vi "Main.vi"(8 "error in (no error)":errorcluster, 11 "ModuleAdmin":refnum<class "ModuleAdmin.lvclass">) -> ()   [LabVIEW 2018, in "ScopePlugins.lvlib"]
uses:
  ScopePlugins.lvlib
  <userlib>/NIST/ModuleAdminLib/ModuleAdmin/ModuleAdmin.lvclass
  C:/Program Files (x86)/National Instruments/LabVIEW 2018/user.lib/NIST/ModuleAdminLib/ModuleAdminBase/ModuleAdminBase.lvclass
  Shared/TypeDefs/QueueNames.ctl
  ScopePluginBaseClass/ScopePluginsBase.lvclass
  C:/Program Files (x86)/National Instruments/LabVIEW 2018/user.lib/NIST/BaseClasses/BasePlugin_class/BasePlugin.lvclass
  Shared/Queue&Messages/EnqueueTypes.ctl
  Shared/Queue&Messages/DequeueTypes.ctl
  ScopeShared/clStopArgument.ctl
  <userlib>/NIST/ModuleAdminLib/ModuleAdmin/ModuleAdmin.lvclass/ModuleAdmin.ctl
  ScopePluginBaseClass/ScopePluginsBase.lvclass/ScopePluginsBase.ctl
  <userlib>/NIST/BaseClasses/BasePlugin_class/BasePlugin.lvclass/BasePlugin.ctl
  InfiniiumClass/Typedefs/ExtAcquisition.ctl
  ScopeShared/Sync.ctl
  <vilib>/Utility/error.llb/DialogType.ctl
  <userlib>/NIST/ModuleAdminLib/ModuleAdmin/Accessors/Read ShowPanel_.vi
  ScopePluginBaseClass/Accessors/Write ModuleID.vi
  ScopePluginBaseClass/Accessors/Read ModuleID.vi
  <userlib>/NIST/ModuleAdminLib/ModuleAdmin/Accessors/Write ShowPanel_.vi
  <userlib>/NIST/BaseClasses/BasePlugin_class/Accessors/Read PluginIniFilePath.vi
  ScopePluginBaseClass/Accessors/Write Sync.vi
  <userlib>/NIST/ModuleAdminLib/ModuleAdmin/Accessors/Read CloneRegRef.vi
  <extravilib>/ChannelInstances/Tag-bool/Read With Abort.vi
  <extravilib>/ChannelInstances/Tag-bool/Write With Abort.vi
  <extravilib>/ChannelInstances/Tag-bool/Instantiate.vi
  <extravilib>/ChannelInstances/Tag-bool/EndpointRead.vi
  <vilib>/Utility/error.llb/Error Cluster From Error Code.vi
  <extravilib>/ChannelInstances/Tag-bool/Endpoint.vi
  <vilib>/ErrorRing/Error Ring.xnode
  <userlib>/NIST/ModuleAdminLib/CloneRegistration/CloneRegistration.lvclass
  ScopeShared/ScopeShared.lvlib
  <userlib>/NIST/ModuleAdminLib/ModuleAdmin.lvlib
  <userlib>/NIST/BaseClasses/Object_class/BaseObject.lvclass
  InfiniiumClass/Infiniium.lvclass
  <extravilib>/ChannelInstances/Tag-bool.lvlib
panel:
  out "EH Loop":i32
  out "QMH Loop":i32
  out "WA Loop":i32
  out "error out":errorcluster
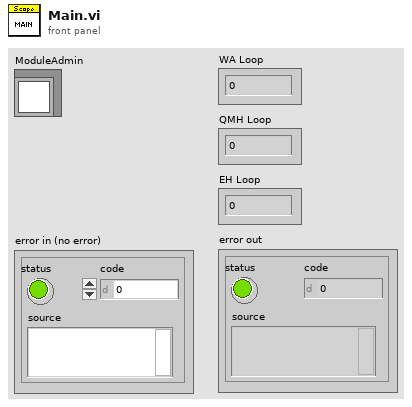
[diagram p1: front panel]
types:
  T1 = typedef "ScopePlugins.lvlib/EnqueueTypes.ctl" = enum16{"LossyEnqueue", "EnqueueAtFront", "Enqueue"}
  T2 = typedef "ScopePlugins.lvlib/QueueNames.ctl" = enum16{"QMH", "Class ", "MA"}
  T3 = typedef "ScopeShared.lvlib/clRequestEvents.ctl" = cluster{"StopRequest":refnum<user-event>, "PathToINI":refnum<user-event>, " LoadPlugin":refnum<user-event>, "ShowPanel":refnum<user-event>, "Abort":refnum<user-event>, "SetAcquisition":refnum<user-event>, "SetChannel":refnum<user-event>, "SetTrigger":refnum<user-event>, "GetAcquisition":refnum<user-event>, "GetChannel":refnum<user-event>, "GetTrigger":refnum<user-event>, "FetchWaveform":refnum<user-event>, "InitAcquisition":refnum<user-event>, "ReadWaveform":refnum<user-event>, "GetHandle":refnum<user-event>, "SetHandle":refnum<user-event>, "GetModel":refnum<user-event>, "SetModel":refnum<user-event>, "ConfigAquisition":refnum<user-event>, "ConfigChannels":refnum<user-event>, "ConfigTrigger":refnum<user-event>, "Initialize":refnum<user-event>, "SetExtAcquisition":refnum<user-event>, "StopAcquisition":refnum<user-event>, "PrefDlg":refnum<user-event>, "Close":refnum<user-event>, "SetSync":refnum<user-event>}
  T4 = typedef "ScopeShared.lvlib/clBroadcastEvents.ctl" = cluster{"DidInit":refnum<user-event>, "StatusUpdate":refnum<user-event>, "ErrorReport":refnum<user-event>, "DidStop":refnum<user-event>, "PathToINI":refnum<user-event>, "Handle":refnum<user-event>, "Model":refnum<user-event>, "Channels":refnum<user-event>, "Acquisition":refnum<user-event>, "Trigger":refnum<user-event>, "ExtAcquisition":refnum<user-event>, "Waveform":refnum<user-event>}
  T5 = typedef "ScopePlugins.lvlib/DequeueTypes.ctl" = enum16{"PreviewQueue", "Dequeue"}
  T6 = typedef "ScopeShared.lvlib/clStopArgument.ctl" = cluster{"Exit via Stop Module Req?":bool, "Wait for Module to stop?":bool, "ModuleAdmin":refnum<class "ModuleAdmin.lvclass">}
  T7 = enum32{"Invalid", "Standard", "Closed", "Hidden", "Minimized", "Maximized"}
  T8 = typedef "ScopePlugins.lvlib/Infiniium.lvclass/ExtAcquisition.ctl" = cluster{"SamplingMode ":enum16{"Real Time", "Equivalent Time", "Segment", "Real Time Peak Detect", "Real Time High Resolution", "Peak Detect Segment", "High Resolution Segment"}, "Interpolation":enum16{"No Interpolation", "sin(x)/x", "linear", "1 Point sin(x)/x", "2 Point sin(x)/x", "4 Point sin(x)/x", "8 Point sin(x)/x", "16 Point sin(x)/x"}, "NumAverages":i32, "EnableAveraging":bool, "Resolution":enum16{"Auto", "Bits 9", "Bits 10", "Bits 11", "Bits 12"}}
  T9 = typedef "ScopeShared.lvlib/Sync.ctl" = cluster{"Handle":string, "SrcTerm":string, "DestTerm":string}
  T10 = typedef "ScopeShared.lvlib/Waveform.ctl" = cluster{"initial x":dbl, "x increment":dbl, "waveform array":dbl[]}
  T11 = typedef "Tag-bool.lvlib/))Channel.ctl" = refnum<queue>
  T12 = typedef "DialogType.ctl" = u16
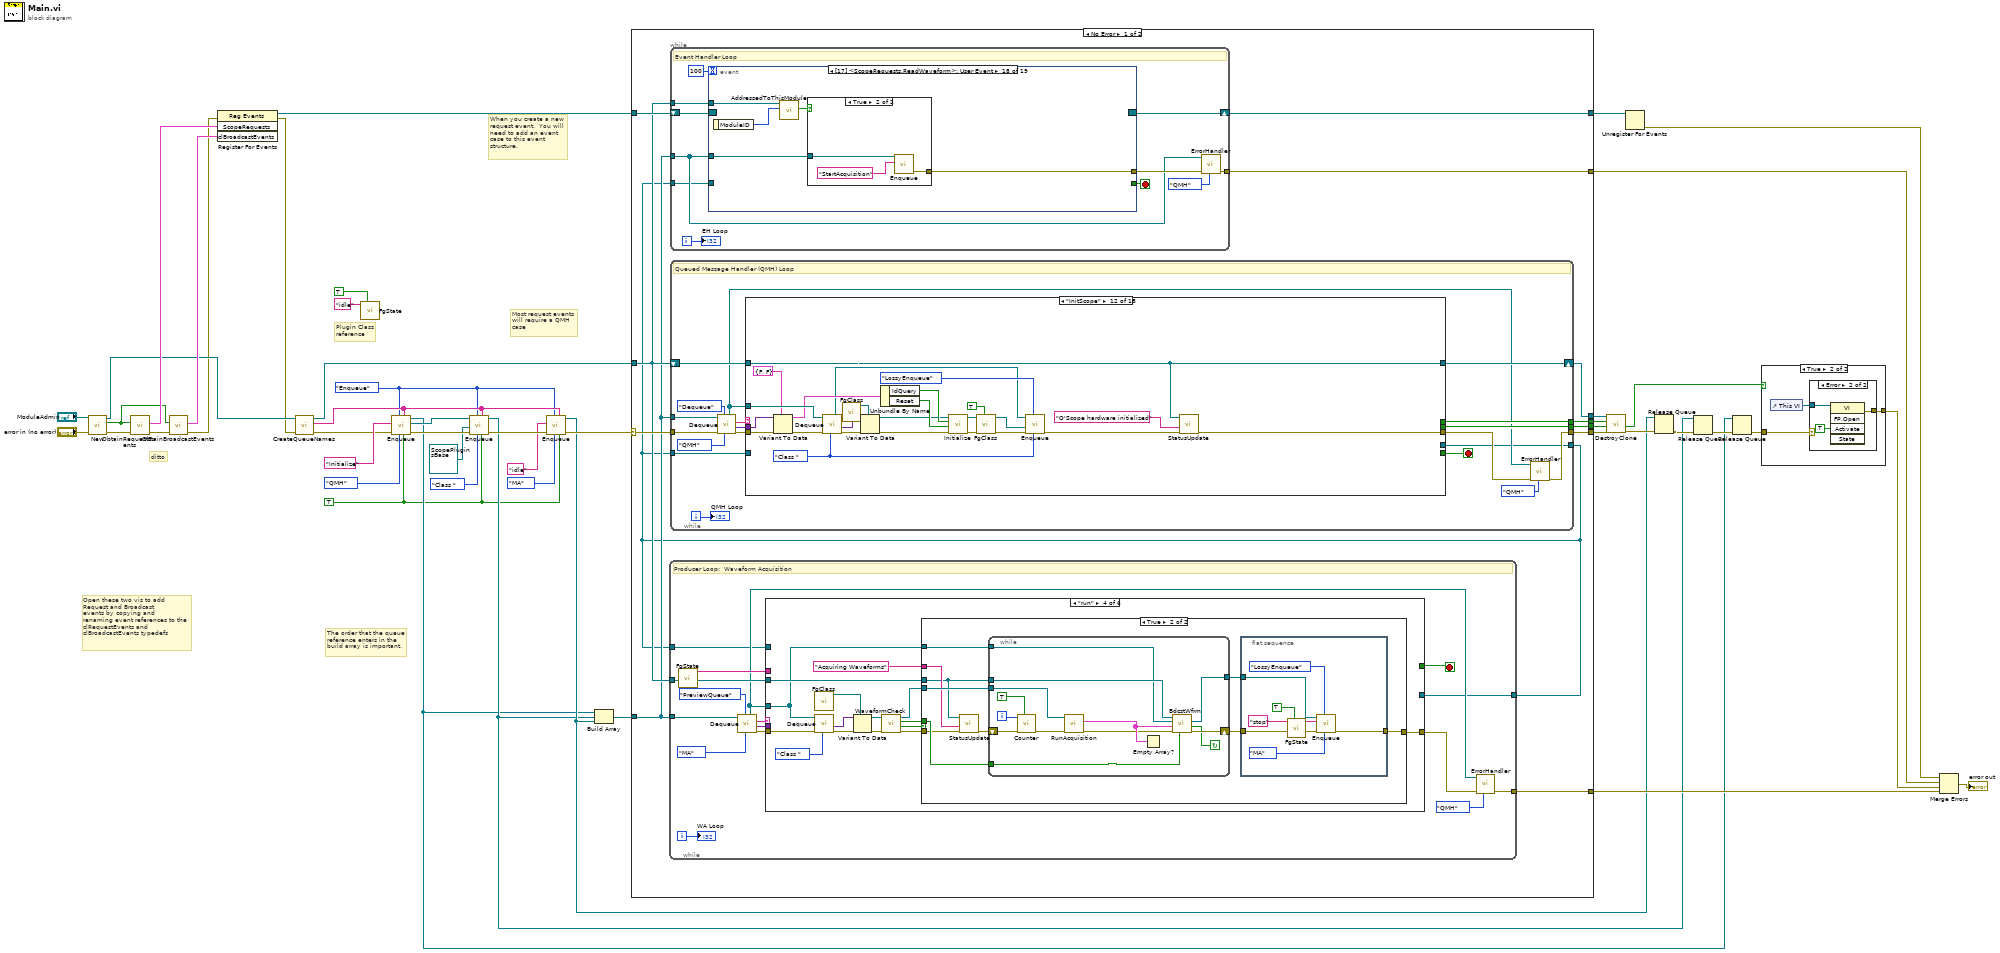
[diagram p0: block diagram]
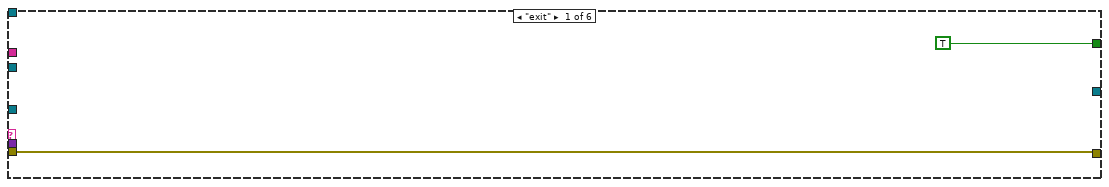
[diagram p2: hidden frame]
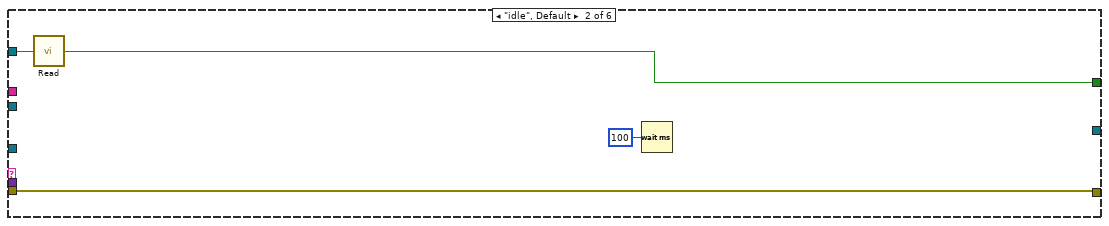
[diagram p3: hidden frame]
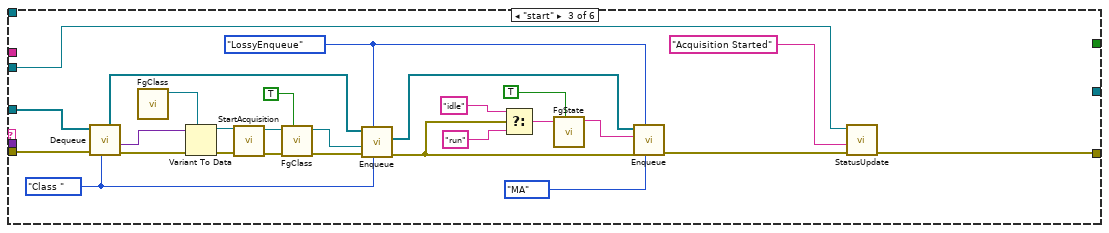
[diagram p4: hidden frame]
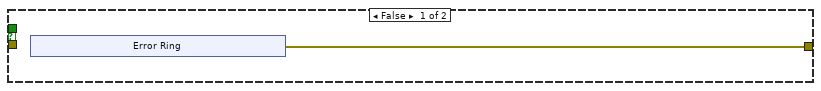
[diagram p5: hidden frame]
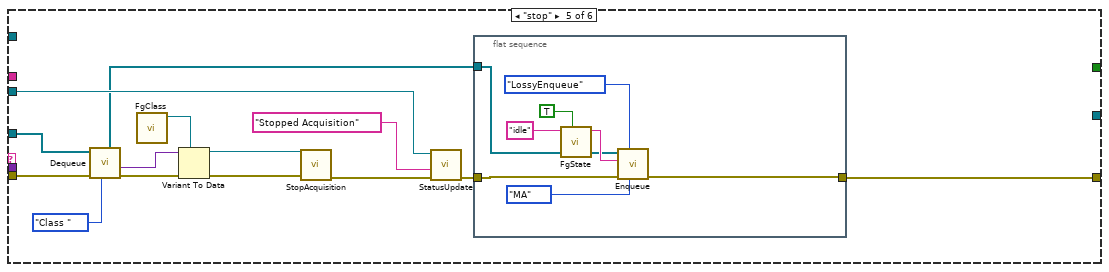
[diagram p6: hidden frame]
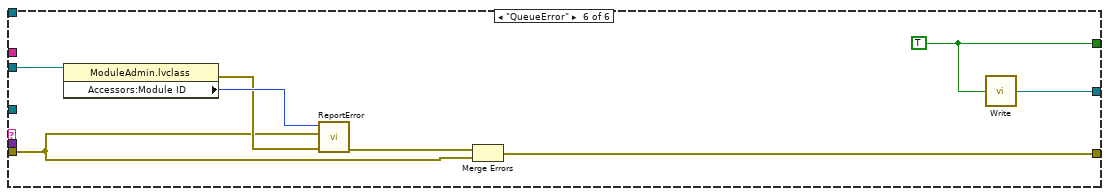
[diagram p7: hidden frame]
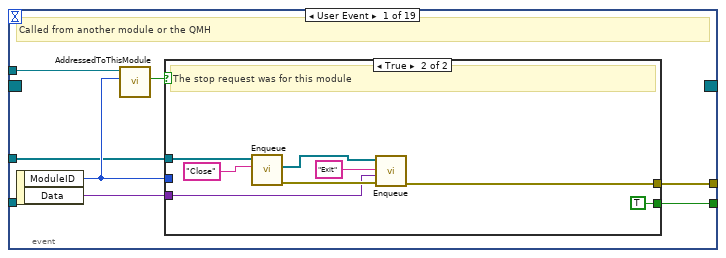
[diagram p8: hidden frame]
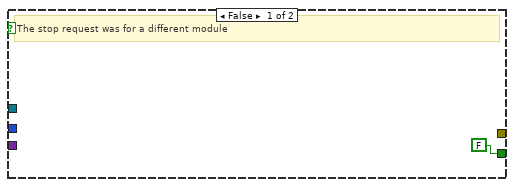
[diagram p9: hidden frame]
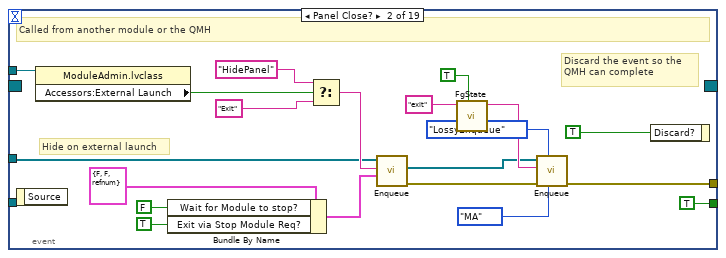
[diagram p10: hidden frame]
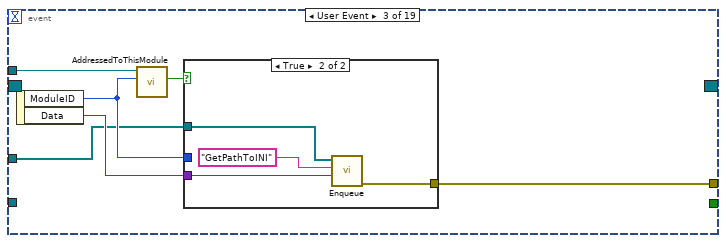
[diagram p11: hidden frame]
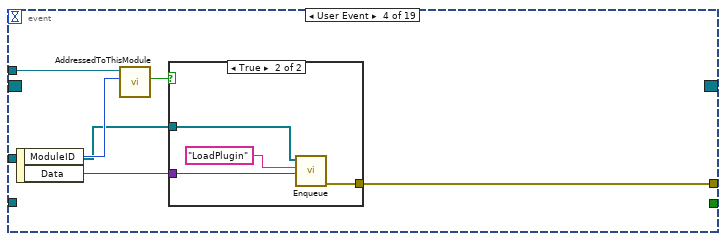
[diagram p13: hidden frame]
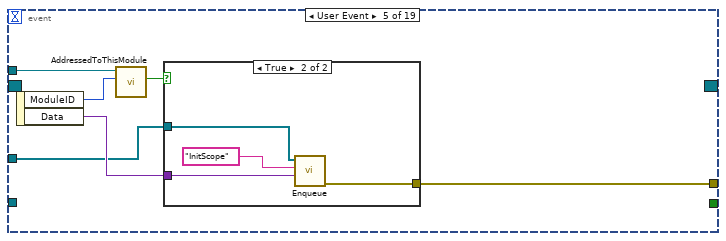
[diagram p15: hidden frame]
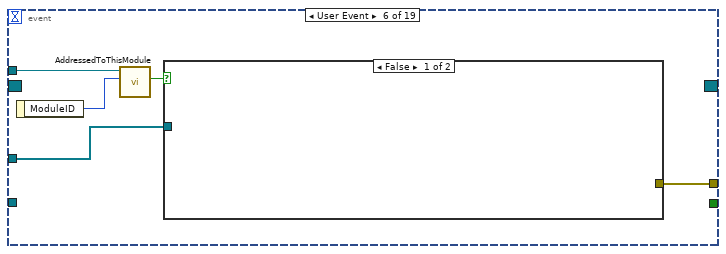
[diagram p17: hidden frame]
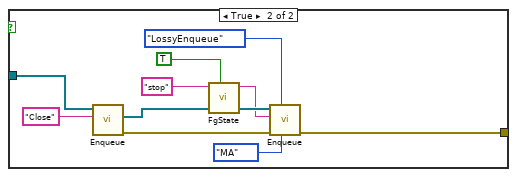
[diagram p18: hidden frame]
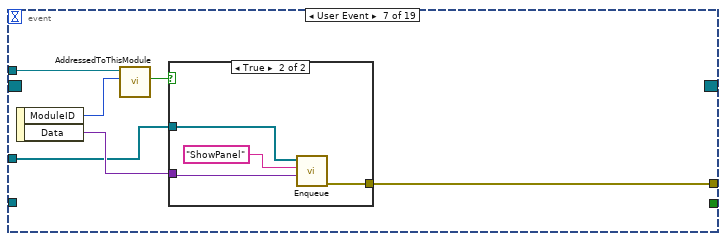
[diagram p19: hidden frame]
diagram:
  w3 = EnqueueTypes."Enqueue" ("EnqueueType (Enqueue)")
  w4 = TRUE ("Frist Call (F)")
  # "The order that the queue\nreference enters in the \nbuild array is important."
  # "Plugin Class\nreference"
  # "Open these two vis to add\nRequest and Broadcast \nevents by copying and \nrenaming event references to the \nclRequestEvents and \nclBroadcastEvents typedefs"
  # "ditto"
  # "Most request events\nwill require a QMH\ncase"
  # "When you create a new request event.  You will need to add an event case to this event structure."
  n1 = call <userlib>:"New.vi"("error in (no error)"="error in (no error)", "ModuleAdmin"="ModuleAdmin") -> ("error out"=w45:errorcluster, "First?"=w43:bool, "ModuleAdmin"=w28:refnum<class "ModuleAdmin.lvclass">)  [unwired: 6 in, 1 out]
  n2 = call "ObtainRequestEvents.vi"("error in (no error)"=w45, "CreateNew (F)"=w43) -> ("error out"=w42:errorcluster, "ScopeRequests"=w44:T3)  [unwired: 8 in]
  n3 = call "ObtainBroadcastEvents.vi"("error in (no error)"=w42, "CreateNew? (F)"=w43) -> ("error out"=w25:errorcluster, "clBroadcastEvents"=w41:T4)  [unwired: 8 in]
  n4 = register-events(error in=w25, w44, w41) -> (reference out=w40:refnum<event-registration>, error out=w26:errorcluster)  [unwired: 1 in]
  n5 = call "CreateQueueNames.vi"("error in (no error)"=w26, "ModuleAdmin In"=w28) -> ("error out"=w19:errorcluster, "QueueNames Out"=w9:string[], "ModuleAdmin Out"=w27:refnum<class "ModuleAdmin.lvclass">)  [unwired: 7 in]
  n6 = call "FgState.vi"("Set (F)"=TRUE, "State In"="idle") -> ()  [unwired: 9 in, 1 out]
  n7 = call "Enqueue.vi"("Frist Call (F)"=w4, "QueueNames In"=w9, "EnqueueType (QMH)"=QueueNames."QMH", "EnqueueType (Enqueue)"=w3, "error in (no error)"=w19, "Message"="Initialize") -> ("error out"=w18:errorcluster, "Queue Array Reference Out"=w16:refnum<queue>[], "MessageQueue"=w6:refnum<queue>)  [unwired: 3 in]
  n8 = call "Enqueue.vi"("Frist Call (F)"=w4, "QueueNames In"=w9, "EnqueueType (QMH)"=QueueNames."Class ", "EnqueueType (Enqueue)"=w3, "error in (no error)"=w18, "Message Data"=refnum<class "ScopePluginsBase.lvclass"> refnum ("MyPlugins.lvlib:MyPluginsBase.lvclass"), "Queue Array Reference In"=w16) -> ("error out"=w15:errorcluster, "MessageQueue"=w7:refnum<queue>)  [unwired: 2 in, 1 out]
  n9 = call "Enqueue.vi"("Frist Call (F)"=w4, "QueueNames In"=w9, "EnqueueType (QMH)"=QueueNames."MA", "EnqueueType (Enqueue)"=w3, "error in (no error)"=w15, "Message"="idle") -> ("error out"=w14:errorcluster, "MessageQueue"=w8:refnum<queue>)  [unwired: 3 in, 1 out]
  n10 = Build Array(w6, w7, w8) -> (w5:refnum<queue>[])
  n11 = case shown="No Error" w14 {
    selector: w14 -> [w52 w773]
    tunnel: w27 -> [w51 w771]
    tunnel: [w59 w767] -> w39
    tunnel: w40 -> [w58 w766]
    tunnel: [w57 w770] -> w37
    tunnel: [w56 _] -> w36
    tunnel: [w55 _] -> w35
    tunnel: [w54 w767] -> w11
    tunnel: [w53 w767] -> w30
    tunnel: w5 -> [w50 _]
    tunnel: [w48 w766] -> w2
    frame No Error {
      n12 = while {
        tunnel: [w72] -> w53
        tunnel: w50 -> [w67]
        tunnel: w51 -> [w64]
        tunnel: [w61] -> w49
        tunnel: w49 -> [w60]
        i -> [w63]
        stop <- w74 stop-if-true
        # "Producer Loop:  Waveform Acquisition"
        n13 = call "FgState.vi"() -> ("State Out"=w75:string)  [unwired: 11 in]
        n14 = call "Dequeue.vi"("EnqueueType (QMH)"=QueueNames."MA", "DequeueType (PreviewQueue)"=DequeueTypes."PreviewQueue", "Queue Array Reference In"=w67) -> ("error out"=w71:errorcluster, "Message Data"=w69:variant, "Message"=w70:string, "Queue Array Reference Out"=w62:refnum<queue>[])  [unwired: 4 in, 1 out]
        n15 = case shown="\"run\"" w70 {
          tunnel: [TRUE w78 _ _ _ w183] -> w74
          tunnel: [w76 w80 w82 w122 w170 w184] -> w73
          tunnel: w71 -> [w76 w80 w100 w112 w168 w186]
          tunnel: w69 -> [_ _ _ _ _ _]
          tunnel: w64 -> [_ _ w83 w121 w169 w185]
          tunnel: w75 -> [_ _ _ _ _ _]
          tunnel: w62 -> [_ _ w87 w108 w161 _]
          tunnel: [_ _ _ _ _ w182] -> w61
          tunnel: w60 -> [_ w79 _ _ _ _]
          frame "exit" {
          }
          frame "idle", Default {
            n16 = call <extravilib>:"Read.vi"("channel"=w79) -> ("element"=w78:bool)  [unwired: 1 in, 1 out]
            n17 = Wait (ms)(milliseconds to wait=u32 100) -> ()  [unwired: 1 out]
          }
          frame "start" {
            w98 = QueueNames."Class " ("EnqueueType (QMH)")
            w86 = EnqueueTypes."LossyEnqueue" ("EnqueueType (Enqueue)")
            n18 = call "Dequeue.vi"("EnqueueType (QMH)"=w98, "error in (no error)"=w100, "Queue Array Reference In"=w87) -> ("error out"=w103:errorcluster, "Message Data"=w102:variant, "Queue Array Reference Out"=w88:refnum<queue>[])  [unwired: 4 in, 2 out]
            n19 = call "FgClass.vi"() -> ("Class Out"=w101:refnum<class "ScopePluginsBase.lvclass">)  [unwired: 11 in]
            n20 = Variant To Data(error in=w103, type=w101, Variant=w102) -> (data=w97:refnum<class "ScopePluginsBase.lvclass">, error out=w99:errorcluster)
            n21 = call-dynamic "StartAcquisition.vi"("error in (no error)"=w99, "ScopePluginsBase in"=w97) -> ("error out"=w104:errorcluster, "ScopePluginsBase out"=w90:refnum<class "ScopePluginsBase.lvclass">)  [unwired: 8 in]
            n22 = call "FgClass.vi"("Set (F)"=TRUE, "Class In"=w90) -> ("Class Out"=w89:refnum<class "ScopePluginsBase.lvclass">)  [unwired: 9 in]
            n23 = call "Enqueue.vi"("EnqueueType (QMH)"=w98, "EnqueueType (Enqueue)"=w86, "error in (no error)"=w104, "Message Data"=w89, "Queue Array Reference In"=w88) -> ("error out"=w96:errorcluster, "Queue Array Reference Out"=w95:refnum<queue>[])  [unwired: 4 in, 1 out]
            n24 = Select(t="idle" ("State In"), s=w96, f="run") -> (s? t:f=w94:string)
            n25 = call "FgState.vi"("Set (F)"=TRUE, "State In"=w94) -> ("State Out"=w92:string)  [unwired: 9 in]
            n26 = call "Enqueue.vi"("EnqueueType (QMH)"=QueueNames."MA", "EnqueueType (Enqueue)"=w86, "error in (no error)"=w96, "Message"=w92, "Queue Array Reference In"=w95) -> ("error out"=w84:errorcluster)  [unwired: 4 in, 2 out]
            n27 = call "StatusUpdate.vi"("error in (no error)"=w84, "Status"="Acquisition Started", "ModuleAdmin"=w83) -> ("error out"=w82:errorcluster)  [unwired: 8 in]
          }
          frame "run" {
            n28 = call "FgClass.vi"() -> ("Class Out"=w110:refnum<class "ScopePluginsBase.lvclass">)  [unwired: 11 in]
            n29 = call "Dequeue.vi"("EnqueueType (QMH)"=QueueNames."Class ", "error in (no error)"=w112, "Queue Array Reference In"=w108) -> ("error out"=w115:errorcluster, "Message Data"=w114:variant)  [unwired: 4 in, 3 out]
            n30 = Variant To Data(error in=w115, type=w110, Variant=w114) -> (data=w109:refnum<class "ScopePluginsBase.lvclass">, error out=w111:errorcluster)
            n31 = call "WaveformCheck.vi"("error in (no error)"=w111, "Class In"=w109) -> ("error out"=w116:errorcluster, "Run?"=w118:bool, "Continuous"=w119:bool, "Class Out"=w117:refnum<class "ScopePluginsBase.lvclass">)  [unwired: 6 in]
            n32 = case shown="True" w118 {
              tunnel: [w123 w136] -> w122
              tunnel: w117 -> [_ w138]
              tunnel: w119 -> [_ w137]
              tunnel: w116 -> [_ w135]
              tunnel: w121 -> [_ w131]
              tunnel: "Acquiring Waveforms" ("Status") -> [_ w132]
              tunnel: w108 -> [_ w130]
              frame False {
                n33 = xnode "Error Ring"() -> ("error out"=w123:errorcluster)
              }
              frame True {
                n34 = call "StatusUpdate.vi"("error in (no error)"=w135, "Status"=w132, "ModuleAdmin"=w131) -> ("error out"=w134:errorcluster)  [unwired: 8 in]
                n35 = while {
                  tunnel: w138 -> [w151]
                  tunnel: w137 -> [w139]
                  shift-right: [w150] -> w133
                  shift-left: w134 -> [w148]
                  tunnel: w131 -> [w144]
                  tunnel: w130 -> [w141]
                  tunnel: [w143] -> w129
                  i -> [w146]
                  stop <- w140 continue-if-true
                  n36 = call "Counter.vi"("Set (f)"=TRUE, "error in (no error)"=w148, "Counter In"=w146) -> ("error out"=w147:errorcluster)  [unwired: 7 in, 1 out]
                  n37 = call-dynamic "RunAcquisition.vi"("error in (no error)"=w147, "ScopePluginsBase in"=w151) -> ("error out"=w142:errorcluster, "Waveforms"=w149:T10[])  [unwired: 7 in, 1 out]
                  n38 = Empty Array?(array=w149) -> ()  [unwired: 1 out]
                  n39 = call "BdcstWfrm.vi"("Continuous"=w139, "error in (no error)"=w142, "Waveforms"=w149, "Queue Array Reference In"=w141, "ModuleAdmin"=w144) -> ("error out"=w150:errorcluster, "Continue"=w140:bool, "Queue Array Reference Out"=w143:refnum<queue>[])  [unwired: 4 in]
                }
                n40 = flat-sequence {
                  tunnel: w133 -> [w156]
                  tunnel: [w155] -> w136
                  tunnel: w129 -> [w152]
                  frame #0 {
                    n41 = call "FgState.vi"("Set (F)"=TRUE, "State In"="stop") -> ("State Out"=w153:string)  [unwired: 9 in]
                    n42 = call "Enqueue.vi"("EnqueueType (QMH)"=QueueNames."MA", "EnqueueType (Enqueue)"=EnqueueTypes."LossyEnqueue", "error in (no error)"=w156, "Message"=w153, "Queue Array Reference In"=w152) -> ("error out"=w155:errorcluster)  [unwired: 4 in, 2 out]
                  }
                }
              }
            }
          }
          frame "stop" {
            n43 = call "Dequeue.vi"("EnqueueType (QMH)"=QueueNames."Class ", "error in (no error)"=w168, "Queue Array Reference In"=w161) -> ("error out"=w167:errorcluster, "Message Data"=w166:variant, "Queue Array Reference Out"=w160:refnum<queue>[])  [unwired: 4 in, 2 out]
            n44 = call "FgClass.vi"() -> ("Class Out"=w163:refnum<class "ScopePluginsBase.lvclass">)  [unwired: 11 in]
            n45 = Variant To Data(error in=w167, type=w163, Variant=w166) -> (data=w162:refnum<class "ScopePluginsBase.lvclass">, error out=w165:errorcluster)
            n46 = call-dynamic "StopAcquisition.vi"("error in (no error)"=w165, "ScopePluginsBase in"=w162) -> ("error out"=w172:errorcluster)  [unwired: 8 in, 1 out]
            n47 = call "StatusUpdate.vi"("error in (no error)"=w172, "Status"="Stopped Acquisition", "ModuleAdmin"=w169) -> ("error out"=w171:errorcluster)  [unwired: 8 in]
            n48 = flat-sequence {
              tunnel: w171 -> [w179]
              tunnel: [w178] -> w170
              tunnel: w160 -> [w174]
              frame #0 {
                n49 = call "FgState.vi"("Set (F)"=TRUE, "State In"="idle") -> ("State Out"=w175:string)  [unwired: 9 in]
                n50 = call "Enqueue.vi"("EnqueueType (QMH)"=QueueNames."MA", "EnqueueType (Enqueue)"=EnqueueTypes."LossyEnqueue", "error in (no error)"=w179, "Message"=w175, "Queue Array Reference In"=w174) -> ("error out"=w178:errorcluster)  [unwired: 4 in, 2 out]
              }
            }
          }
          frame "QueueError" {
            w183 = TRUE ("Boolean")
            n51 = property class="ModuleAdmin.lvclass"(reference=w185) -> (error out=w188:errorcluster, "Accessors:Module ID"=w189:i32)  [unwired: 1 in, 1 out]
            n52 = call "ReportError.vi"("error in (no error)"=w188, "ErrorReported"=w186, "ModuleID"=w189) -> ("error out"=w187:errorcluster)  [unwired: 8 in]
            n53 = Merge Errors(w187, w186) -> (w184:errorcluster)
            n54 = call <extravilib>:"Write.vi"("element"=w183) -> ("channel"=w182:T11)  [unwired: 1 out]
          }
        }
        n55 = call "ErrorHandler.vi"("EnqueueType (QMH)"=QueueNames."QMH", "error in (no error)"=w73, "Queue Array Reference In"=w62) -> ("error out"=w72:errorcluster)  [unwired: 8 in]
        "WA Loop" <- w63
      }
      n56 = while {
        shift-right: [w198] -> w48
        shift-left: w58 -> [w199]
        tunnel: w51 -> [w197]
        tunnel: [w195] -> w54
        tunnel: w50 -> [w194]
        tunnel: w49 -> [w190]
        i -> [w192]
        stop <- w200 stop-if-true
        # "Event Handler Loop"
        n57 = event shown="[17] <ScopeRequests.ReadWaveform>: User Event" {
          selector: w199 -> [_ _ _ _ _ _ _ _ _ _ _ _ _ _ _ _ _ _ _]
          dyn-events: [_ _ _ _ _ _ _ _ _ _ _ _ _ _ _ _ _ _ _] -> w198
          timeout: 100 -> [_ _ _ _ _ _ _ _ _ _ _ _ _ _ _ _ _ _ _]
          tunnel: [w204 TRUE _ _ _ _ _ _ _ _ _ _ _ _ _ _ _ _ w395] -> w200
          tunnel: w197 -> [w207 w231 w238 w251 w261 w270 w286 w295 w304 w316 w326 w336 w345 w353 w362 w372 w382 w391 _]
          tunnel: [w203 w222 w237 w248 w258 w267 w283 w291 w301 w313 w323 w333 w341 w349 w359 w369 w379 w388 _] -> w196
          tunnel: w194 -> [w201 w219 w236 w246 w256 w266 w281 _ w300 w311 w321 w331 w342 w350 w357 w367 w377 w387 _]
          tunnel: w190 -> [_ _ _ _ _ _ _ _ _ _ _ _ _ _ _ _ _ _ w396]
          event User Event {
            # "Called from another module or the QMH"
            n58 = event-data() -> ("ModuleID"=w205:i32, "Data"=w202:variant)  [unwired: 1 in]
            n59 = call <userlib>:"AddressedToThisModule.vi"("ModuleID"=w205, "ModuleAdmin"=w207) -> ("AddressedToThisInstance?"=w206:bool)  [unwired: 8 in, 1 out]
            n60 = case shown="True" w206 {
              tunnel: w205 -> [_ _]
              tunnel: [FALSE TRUE] -> w204
              tunnel: [_ w215] -> w203
              tunnel: w202 -> [_ w211]
              tunnel: w201 -> [_ w210]
              frame False {
                # "The stop request was for a different module"
              }
              frame True {
                # "The stop request was for this module"
                n61 = call "Enqueue.vi"("Message"="Close", "Queue Array Reference In"=w210) -> ("error out"=w212:errorcluster, "Queue Array Reference Out"=w209:refnum<queue>[])  [unwired: 7 in, 1 out]
                n62 = call "Enqueue.vi"("error in (no error)"=w212, "Message Data"=w211, "Message"="Exit", "Queue Array Reference In"=w209) -> ("error out"=w215:errorcluster)  [unwired: 5 in, 2 out]
              }
            }
          }
          event Panel Close? {
            w221 = "exit" ("State In")
            # "Hide on external launch"
            # "Discard the event so the QMH can complete"
            # "Called from another module or the QMH"
            n63 = event-data() -> ()  [unwired: 1 in, 1 out]
            n64 = property class="ModuleAdmin.lvclass"(reference=w231) -> ("Accessors:External Launch"=w226:bool)  [unwired: 1 in, 2 out]
            n65 = Bundle By Name(cluster=T6 {"Exit via Stop Module Req?"=FALSE, "Wait for Module to stop?"=FALSE, "ModuleAdmin"=refnum} ("Stop Argument"), "Wait for Module to stop?"=FALSE, "Exit via Stop Module Req?"=TRUE) -> (w232:T6)
            n66 = Select(t="HidePanel", s=w226, f="Exit" ("Message")) -> (s? t:f=w228:string)
            n67 = call "Enqueue.vi"("Message Data"=w232, "Message"=w228, "Queue Array Reference In"=w219) -> ("error out"=w223:errorcluster, "Queue Array Reference Out"=w220:refnum<queue>[])  [unwired: 6 in, 1 out]
            n68 = call "FgState.vi"("Set (F)"=TRUE, "State In"=w221) -> ()  [unwired: 9 in, 1 out]
            n69 = call "Enqueue.vi"("EnqueueType (QMH)"=QueueNames."MA", "EnqueueType (Enqueue)"=EnqueueTypes."LossyEnqueue", "error in (no error)"=w223, "Message"=w221, "Queue Array Reference In"=w220) -> ("error out"=w222:errorcluster)  [unwired: 4 in, 2 out]
            n70 = event-data("Discard?"=TRUE) -> ()  [unwired: 1 in, 1 out]
          }
          event User Event {
            n71 = event-data() -> ("ModuleID"=w239:i32, "Data"=w240:variant)  [unwired: 1 in]
            n72 = call <userlib>:"AddressedToThisModule.vi"("ModuleID"=w239, "ModuleAdmin"=w238) -> ("AddressedToThisInstance?"=w241:bool)  [unwired: 8 in, 1 out]
            n73 = case shown="True" w241 {
              tunnel: w239 -> [_ _]
              tunnel: [_ w245] -> w237
              tunnel: w240 -> [_ w243]
              tunnel: w236 -> [_ w242]
              frame False {
                # "The stop request was for a different module"
              }
              frame True {
                # "The stop request was for this module"
                n74 = call "Enqueue.vi"("Message Data"=w243, "Message"="GetPathToINI", "Queue Array Reference In"=w242) -> ("error out"=w245:errorcluster)  [unwired: 6 in, 2 out]
              }
            }
          }
          event User Event {
            n75 = event-data() -> ("ModuleID"=w250:i32, "Data"=w247:variant)  [unwired: 1 in]
            n76 = call <userlib>:"AddressedToThisModule.vi"("ModuleID"=w250, "ModuleAdmin"=w251) -> ("AddressedToThisInstance?"=w249:bool)  [unwired: 8 in, 1 out]
            n77 = case shown="True" w249 {
              tunnel: [_ w253] -> w248
              tunnel: w247 -> [_ w254]
              tunnel: w246 -> [_ w252]
              frame False {
              }
              frame True {
                n78 = call "Enqueue.vi"("Message Data"=w254, "Message"="LoadPlugin", "Queue Array Reference In"=w252) -> ("error out"=w253:errorcluster)  [unwired: 6 in, 2 out]
              }
            }
          }
          event User Event {
            n79 = event-data() -> ("ModuleID"=w260:i32, "Data"=w257:variant)  [unwired: 1 in]
            n80 = call <userlib>:"AddressedToThisModule.vi"("ModuleID"=w260, "ModuleAdmin"=w261) -> ("AddressedToThisInstance?"=w259:bool)  [unwired: 8 in, 1 out]
            n81 = case shown="True" w259 {
              tunnel: [_ w263] -> w258
              tunnel: w257 -> [_ w264]
              tunnel: w256 -> [_ w262]
              frame False {
              }
              frame True {
                n82 = call "Enqueue.vi"("Message Data"=w264, "Message"="InitScope", "Queue Array Reference In"=w262) -> ("error out"=w263:errorcluster)  [unwired: 6 in, 2 out]
              }
            }
          }
          event User Event {
            n83 = event-data() -> ("ModuleID"=w269:i32)  [unwired: 1 in]
            n84 = call <userlib>:"AddressedToThisModule.vi"("ModuleID"=w269, "ModuleAdmin"=w270) -> ("AddressedToThisInstance?"=w268:bool)  [unwired: 8 in, 1 out]
            n85 = case shown="False" w268 {
              tunnel: [_ w277] -> w267
              tunnel: w266 -> [_ w275]
              frame False {
              }
              frame True {
                n86 = call "Enqueue.vi"("Message"="Close", "Queue Array Reference In"=w275) -> ("error out"=w278:errorcluster, "Queue Array Reference Out"=w273:refnum<queue>[])  [unwired: 7 in, 1 out]
                n87 = call "FgState.vi"("Set (F)"=TRUE, "State In"="stop") -> ("State Out"=w272:string)  [unwired: 9 in]
                n88 = call "Enqueue.vi"("EnqueueType (QMH)"=QueueNames."MA", "EnqueueType (Enqueue)"=EnqueueTypes."LossyEnqueue", "error in (no error)"=w278, "Message"=w272, "Queue Array Reference In"=w273) -> ("error out"=w277:errorcluster)  [unwired: 4 in, 2 out]
              }
            }
          }
          event User Event {
            n89 = event-data() -> ("ModuleID"=w285:i32, "Data"=w282:variant)  [unwired: 1 in]
            n90 = call <userlib>:"AddressedToThisModule.vi"("ModuleID"=w285, "ModuleAdmin"=w286) -> ("AddressedToThisInstance?"=w284:bool)  [unwired: 8 in, 1 out]
            n91 = case shown="True" w284 {
              tunnel: [_ w288] -> w283
              tunnel: w282 -> [_ w289]
              tunnel: w281 -> [_ w287]
              frame False {
              }
              frame True {
                n92 = call "Enqueue.vi"("Message Data"=w289, "Message"="ShowPanel", "Queue Array Reference In"=w287) -> ("error out"=w288:errorcluster)  [unwired: 6 in, 2 out]
              }
            }
          }
          event User Event {
            n93 = event-data() -> ("ModuleID"=w294:i32, "Data"=w292:variant)  [unwired: 1 in]
            n94 = call <userlib>:"AddressedToThisModule.vi"("ModuleID"=w294, "ModuleAdmin"=w295) -> ("AddressedToThisInstance?"=w293:bool)  [unwired: 8 in, 1 out]
            n95 = case shown="True" w293 {
              tunnel: w292 -> [_ _]
              tunnel: [_ w296] -> w291
              frame False {
              }
              frame True {
                n96 = call "FgClass.vi"() -> ("Class Out"=w299:refnum<class "ScopePluginsBase.lvclass">)  [unwired: 11 in]
                n97 = call "ConfigDlg.vi"("ScopePluginsBase in"=w299) -> ("error out"=w296:errorcluster, "ScopePluginsBase out"=w298:refnum<class "ScopePluginsBase.lvclass">)  [unwired: 9 in]
                n98 = call "FgClass.vi"("Set (F)"=TRUE, "Class In"=w298) -> ()  [unwired: 9 in, 1 out]
              }
            }
          }
          event User Event {
            n99 = event-data() -> ("ModuleID"=w303:i32)  [unwired: 1 in]
            n100 = call <userlib>:"AddressedToThisModule.vi"("ModuleID"=w303, "ModuleAdmin"=w304) -> ("AddressedToThisInstance?"=w302:bool)  [unwired: 8 in, 1 out]
            n101 = case shown="True" w302 {
              tunnel: [_ w309] -> w301
              tunnel: w300 -> [_ w307]
              frame False {
              }
              frame True {
                w308 = "stop" ("State In")
                n102 = call "FgState.vi"("Set (F)"=TRUE, "State In"=w308) -> ()  [unwired: 9 in, 1 out]
                n103 = call "Enqueue.vi"("EnqueueType (QMH)"=QueueNames."MA", "EnqueueType (Enqueue)"=EnqueueTypes."LossyEnqueue", "Message"=w308, "Queue Array Reference In"=w307) -> ("error out"=w309:errorcluster)  [unwired: 5 in, 2 out]
              }
            }
          }
          event User Event {
            n104 = event-data() -> ("ModuleID"=w315:i32, "Data"=w312:variant)  [unwired: 1 in]
            n105 = call <userlib>:"AddressedToThisModule.vi"("ModuleID"=w315, "ModuleAdmin"=w316) -> ("AddressedToThisInstance?"=w314:bool)  [unwired: 8 in, 1 out]
            n106 = case shown="True" w314 {
              tunnel: [_ w318] -> w313
              tunnel: w312 -> [_ w319]
              tunnel: w311 -> [_ w317]
              frame False {
              }
              frame True {
                n107 = call "Enqueue.vi"("Message Data"=w319, "Message"="Unhandled Event", "Queue Array Reference In"=w317) -> ("error out"=w318:errorcluster)  [unwired: 6 in, 2 out]
              }
            }
          }
          event User Event {
            n108 = event-data() -> ("ModuleID"=w325:i32, "Data"=w322:variant)  [unwired: 1 in]
            n109 = call <userlib>:"AddressedToThisModule.vi"("ModuleID"=w325, "ModuleAdmin"=w326) -> ("AddressedToThisInstance?"=w324:bool)  [unwired: 8 in, 1 out]
            n110 = case shown="True" w324 {
              tunnel: [_ w327] -> w323
              tunnel: w321 -> [_ w330]
              tunnel: w322 -> [_ w328]
              frame False {
              }
              frame True {
                n111 = call "Enqueue.vi"("Message Data"=w328, "Message"="ConfigAcquisition", "Queue Array Reference In"=w330) -> ("error out"=w327:errorcluster)  [unwired: 6 in, 2 out]
              }
            }
          }
          event User Event {
            n112 = event-data() -> ("ModuleID"=w335:i32, "Data"=w332:variant)  [unwired: 1 in]
            n113 = call <userlib>:"AddressedToThisModule.vi"("ModuleID"=w335, "ModuleAdmin"=w336) -> ("AddressedToThisInstance?"=w334:bool)  [unwired: 8 in, 1 out]
            n114 = case shown="True" w334 {
              tunnel: [_ w337] -> w333
              tunnel: w331 -> [_ w340]
              tunnel: w332 -> [_ w338]
              frame False {
              }
              frame True {
                n115 = call "Enqueue.vi"("Message Data"=w338, "Message"="SetExtAquisition", "Queue Array Reference In"=w340) -> ("error out"=w337:errorcluster)  [unwired: 6 in, 2 out]
              }
            }
          }
          event User Event {
            n116 = event-data() -> ("ModuleID"=w344:i32)  [unwired: 1 in]
            n117 = call <userlib>:"AddressedToThisModule.vi"("ModuleID"=w344, "ModuleAdmin"=w345) -> ("AddressedToThisInstance?"=w343:bool)  [unwired: 8 in, 1 out]
            n118 = case shown="True" w343 {
              tunnel: [_ w348] -> w341
              tunnel: w342 -> [_ w346]
              frame False {
              }
              frame True {
                n119 = call "Enqueue.vi"("Message"="StartAcquisition" ("State In"), "Queue Array Reference In"=w346) -> ("error out"=w348:errorcluster)  [unwired: 7 in, 2 out]
              }
            }
          }
          event User Event {
            n120 = event-data() -> ("ModuleID"=w352:i32)  [unwired: 1 in]
            n121 = call <userlib>:"AddressedToThisModule.vi"("ModuleID"=w352, "ModuleAdmin"=w353) -> ("AddressedToThisInstance?"=w351:bool)  [unwired: 8 in, 1 out]
            n122 = case shown="True" w351 {
              tunnel: [_ w356] -> w349
              tunnel: w350 -> [_ w354]
              frame False {
              }
              frame True {
                n123 = call "Enqueue.vi"("Message"="StopAcquisition" ("State In"), "Queue Array Reference In"=w354) -> ("error out"=w356:errorcluster)  [unwired: 7 in, 2 out]
              }
            }
          }
          event User Event {
            n124 = event-data() -> ("ModuleID"=w361:i32, "Data"=w358:variant)  [unwired: 1 in]
            n125 = call <userlib>:"AddressedToThisModule.vi"("ModuleID"=w361, "ModuleAdmin"=w362) -> ("AddressedToThisInstance?"=w360:bool)  [unwired: 8 in, 1 out]
            n126 = case shown="True" w360 {
              tunnel: [_ w363] -> w359
              tunnel: w357 -> [_ w366]
              tunnel: w358 -> [_ w364]
              frame False {
              }
              frame True {
                n127 = call "Enqueue.vi"("Message Data"=w364, "Message"="ConfigTrigger", "Queue Array Reference In"=w366) -> ("error out"=w363:errorcluster)  [unwired: 6 in, 2 out]
              }
            }
          }
          event User Event {
            n128 = event-data() -> ("ModuleID"=w371:i32, "Data"=w368:variant)  [unwired: 1 in]
            n129 = call <userlib>:"AddressedToThisModule.vi"("ModuleID"=w371, "ModuleAdmin"=w372) -> ("AddressedToThisInstance?"=w370:bool)  [unwired: 8 in, 1 out]
            n130 = case shown="True" w370 {
              tunnel: [_ w373] -> w369
              tunnel: w367 -> [_ w376]
              tunnel: w368 -> [_ w374]
              frame False {
              }
              frame True {
                n131 = call "Enqueue.vi"("Message Data"=w374, "Message"="ConfigChannels", "Queue Array Reference In"=w376) -> ("error out"=w373:errorcluster)  [unwired: 6 in, 2 out]
              }
            }
          }
          event User Event {
            n132 = event-data() -> ("ModuleID"=w381:i32, "Data"=w378:variant)  [unwired: 1 in]
            n133 = call <userlib>:"AddressedToThisModule.vi"("ModuleID"=w381, "ModuleAdmin"=w382) -> ("AddressedToThisInstance?"=w380:bool)  [unwired: 8 in, 1 out]
            n134 = case shown="True" w380 {
              tunnel: [_ w383] -> w379
              tunnel: w377 -> [_ w386]
              tunnel: w378 -> [_ w384]
              frame False {
              }
              frame True {
                n135 = call "Enqueue.vi"("Message Data"=w384, "Message"="SetSync", "Queue Array Reference In"=w386) -> ("error out"=w383:errorcluster)  [unwired: 6 in, 2 out]
              }
            }
          }
          event User Event {
            n136 = event-data() -> ("ModuleID"=w390:i32)  [unwired: 1 in]
            n137 = call <userlib>:"AddressedToThisModule.vi"("ModuleID"=w390, "ModuleAdmin"=w391) -> ("AddressedToThisInstance?"=w389:bool)  [unwired: 8 in, 1 out]
            n138 = case shown="True" w389 {
              tunnel: [_ w393] -> w388
              tunnel: w387 -> [_ w392]
              frame False {
              }
              frame True {
                n139 = call "Enqueue.vi"("Message"="StartAcquisition", "Queue Array Reference In"=w392) -> ("error out"=w393:errorcluster)  [unwired: 7 in, 2 out]
              }
            }
          }
          event Timeout {
            n140 = event-data() -> ()  [unwired: 1 in, 3 out]
            n141 = call <extravilib>:"Read.vi"("channel"=w396) -> ("element"=w395:bool)  [unwired: 1 in, 1 out]
          }
        }
        n142 = call "ErrorHandler.vi"("EnqueueType (QMH)"=QueueNames."QMH", "error in (no error)"=w196, "Queue Array Reference In"=w194) -> ("error out"=w195:errorcluster)  [unwired: 8 in]
        "EH Loop" <- w192
      }
      n143 = while {
        tunnel: w52 -> [w414]
        tunnel: [w407] -> w59
        tunnel: [w409] -> w56
        tunnel: [w408] -> w55
        shift-right: [w405] -> w57
        shift-left: w51 -> [w410]
        tunnel: w50 -> [w403]
        tunnel: w49 -> [w398]
        tunnel: w49 -> [w397]
        i -> [w400]
        stop <- w415 stop-if-true
        # "Queued Message Handler (QMH) Loop"
        n144 = call "Dequeue.vi"("EnqueueType (QMH)"=QueueNames."QMH", "DequeueType (PreviewQueue)"=DequeueTypes."Dequeue", "error in (no error)"=w414, "Queue Array Reference In"=w403) -> ("error out"=w413:errorcluster, "Message Data"=w411:variant, "Message"=w412:string, "Queue Array Reference Out"=w399:refnum<queue>[])  [unwired: 3 in, 1 out]
        n145 = case shown="\"InitScope\"" w412 {
          selector: w412 -> [_ _ _ _ _ _ _ _ _ _ _ _ _ _ _ _ _ w754]
          tunnel: [_ _ _ _ _ _ _ _ _ _ _ _ _ w693 w699 _ w747 _] -> w415
          tunnel: w410 -> [w441 w458 w472 w478 w542 w563 w581 w597 w619 w623 w632 w659 w670 w697 w702 w721 w742 w757]
          tunnel: [w433 w452 w473 w479 w528 w562 w580 w596 w621 w622 w631 w658 w671 w691 w701 w719 w746 w750] -> w406
          tunnel: w413 -> [w422 w461 w465 w488 w544 w555 w573 w603 w605 w627 w636 w662 w669 w692 w701 w718 w734 w748]
          tunnel: w411 -> [_ w460 _ w490 w545 _ _ w602 _ _ _ w663 w678 _ _ _ w741 _]
          tunnel: [_ _ _ _ _ _ _ _ _ _ _ _ _ _ _ _ w744 _] -> w409
          tunnel: [_ _ _ _ _ _ _ _ _ _ _ _ _ _ _ _ w743 _] -> w408
          tunnel: [w416 w457 w472 w475 w542 w563 w581 w597 w619 w623 w632 w659 w666 w696 w702 w721 w742 w752] -> w405
          tunnel: w399 -> [_ _ w464 w474 w538 w554 w572 w584 w611 w624 w633 w645 _ _ _ w716 w733 _]
          tunnel: [_ _ _ _ _ _ _ _ _ _ _ _ w664 w690 _ _ w732 _] -> w398
          tunnel: w397 -> [_ _ _ _ _ _ _ _ _ _ _ _ _ _ w700 _ _ _]
          frame "Initialize" {
            # "Initialize is always called after ObtainQueue.vi is run"
            n146 = property class="ModuleAdmin.lvclass"(reference=w441, error in=w422) -> (reference out=w425:refnum<class "ModuleAdmin.lvclass">, error out=w421:errorcluster, "Accessors:ShowPanel_"=w432:bool, "Accessors:External Launch"=w424:bool, "Accessors:ModuleName"=w423:string, "Accessors:Module ID"=w417:i32)
            n147 = Compound Arithmetic op=OR(w432, invert w424) -> (w431:bool)
            n148 = Select(t=T7."Standard" ("Front Panel Window:State"), s=w431, f=T7."Hidden" ("Front Panel Window:State")) -> (s? t:f=w426:T7)
            n149 = invoke class="VI" method="FP.Open"(error in=w421, "State"=w426) -> (error out=w419:errorcluster)  [unwired: 3 in, 4 out]
            n150 = call <userlib>:"ModuleName.vi"("Name"=w423, "ModuleID"=w417) -> ("ModuleName"=w436:string)  [unwired: 9 in]
            n151 = property class="VI"(error in=w419, "Front Panel.Title"=w436) -> (reference out=w440:refnum<vi>, error out=w439:errorcluster)  [unwired: 1 in]
            n152 = invoke class="VI" method="FP.Center"(reference=w440, error in=w439) -> (error out=w418:errorcluster)  [unwired: 1 in, 2 out]
            n153 = property class="ScopePluginsBase.lvclass" props=["Accessors:ModuleID", "Accessors:ModuleID"](reference=refnum<class "ScopePluginsBase.lvclass"> refnum ("MyPlugins.lvlib:MyPluginsBase.lvclass"), error in=w418, "Accessors:ModuleID"=w417) -> (reference out=w427:refnum<class "ScopePluginsBase.lvclass">, error out=w420:errorcluster)  [unwired: 1 out]
            n154 = call "FgClass.vi"("Set (F)"=TRUE, "Class In"=w427) -> ()  [unwired: 9 in, 1 out]
            n155 = case shown="True" w424 {
              tunnel: [w442 w448] -> w434
              tunnel: [w443 w445] -> w430
              tunnel: w420 -> [w442 w447]
              tunnel: w425 -> [w443 w444]
              frame False {
              }
              frame True {
                n156 = call <userlib>:"WaitOnModuleSync.vi"("error in (no error)"=w447, "ModuleAdmin"=w444) -> ("error out"=w449:errorcluster, "ModuleAdmin"=w446:refnum<class "ModuleAdmin.lvclass">)  [unwired: 8 in]
                n157 = call <userlib>:"WaitOnEventSync.vi"("error in (no error)"=w449, "ModuleAdmin"=w446) -> ("error out"=w448:errorcluster, "ModuleAdmin"=w445:refnum<class "ModuleAdmin.lvclass">)  [unwired: 8 in]
              }
            }
            n158 = call "DidInit.vi"("Init?"=TRUE, "error in (no error)"=w434, "ModuleAdmin In"=w430) -> ("error out"=w433:errorcluster, "ModuleAdmin Out"=w416:refnum<class "ModuleAdmin.lvclass">)  [unwired: 7 in]
          }
          frame "ShowPanel" {
            n159 = Variant To Data(error in=w461, type=TRUE, Variant=w460) -> (data=w454:bool, error out=w451:errorcluster)
            n160 = property class="ModuleAdmin.lvclass"(reference=w458, error in=w451, "Accessors:ShowPanel_"=w454) -> (reference out=w457:refnum<class "ModuleAdmin.lvclass">, error out=w450:errorcluster)
            n161 = Select(t=T7."Standard" ("Front Panel Window:State"), s=w454, f=T7."Hidden" ("Front Panel Window:State")) -> (s? t:f=w453:T7)
            n162 = property class="VI"(error in=w450, "FP.State"=w453) -> (error out=w452:errorcluster)  [unwired: 1 in, 1 out]
          }
          frame "GetPathToINI" {
            n163 = call "Dequeue.vi"("EnqueueType (QMH)"=QueueNames."Class ", "error in (no error)"=w465, "Queue Array Reference In"=w464) -> ("error out"=w469:errorcluster, "Message Data"=w468:variant)  [unwired: 4 in, 3 out]
            n164 = call "FgClass.vi"() -> ("Class Out"=w467:refnum<class "ScopePluginsBase.lvclass">)  [unwired: 11 in]
            n165 = Variant To Data(error in=w469, type=w467, Variant=w468) -> (data=w462:refnum<class "ScopePluginsBase.lvclass">, error out=w463:errorcluster)
            n166 = property class="ScopePluginsBase.lvclass"(reference=w462, error in=w463) -> (error out=w470:errorcluster, "Accessors:PluginIniFilePath"=w471:path)  [unwired: 1 out]
            n167 = call "PathToINIBroadcast.vi"("error in (no error)"=w470, "PathToINI"=w471, "ModuleAdmin"=w472) -> ("error out"=w473:errorcluster)  [unwired: 8 in]
          }
          frame "LoadPlugin" {
            n168 = Variant To Data(error in=w488, type=path "", Variant=w490) -> (data=w476:path, error out=w487:errorcluster)
            n169 = disable-structure shown="Enabled" {
              disable-tunnel: [w493 w494] -> w477
              disable-tunnel: w476 -> [w491 w494]
              frame Disabled {
                n170 = Current VI's Path() -> (path=w492:path)
                n171 = Build Path(base path=w492, name or relative path=w491) -> (appended path=w493:path)
              }
              frame Enabled {
              }
            }
            n172 = call <userlib>:"GetPathToClass.vi"("error in (no error)"=w487, "configuration file path"=w477) -> ("error IO"=w483:errorcluster, "PathToClass"=w486:path)  [unwired: 8 in]
            n173 = Current VI's Path() -> (path=w485:path)
            n174 = Build Path(base path=w485, name or relative path=w486) -> (appended path=w484:path)
            n175 = call <vilib>:"Check if File or Folder Exists.vi"("error in (no error)"=w483, "path"=w484) -> ("error out"=w480:errorcluster, "file or folder exists?"=w482:bool, "dup path"=w481:path)  [unwired: 7 in]
            n176 = case shown="True" w482 {
              tunnel: w481 -> [w497 w518]
              tunnel: w480 -> [_ w525]
              tunnel: [w496 w520] -> w479
              tunnel: w478 -> [w495 w519]
              tunnel: w476 -> [_ w512]
              tunnel: [w495 w519] -> w475
              tunnel: w474 -> [_ w507]
              frame False {
                n177 = Path To String(path=w497) -> (string=w498:string)
                n178 = xnode "Error Ring"("parameter 0"=w498) -> ("error out"=w496:errorcluster)
              }
              frame True {
                n179 = call-dynamic "LoadClassFromFile.vi"("error in (no error)"=w525, "class path"=w518, "reference in"=refnum<class "ScopePluginsBase.lvclass"> refnum ("MyPlugins.lvlib:MyPluginsBase.lvclass")) -> ("error out"=w516:errorcluster, "reference out"=w517:refnum<class "ScopePluginsBase.lvclass">)  [unwired: 7 in]
                n180 = call-dynamic "GetDefaultParams.vi"("error in (no error)"=w516, "config file path"=w512, "ScopeBase"=w517) -> ("error out"=w510:errorcluster, "ScopeBase"=w515:refnum<class "ScopePluginsBase.lvclass">)  [unwired: 6 in, 1 out]
                n181 = call "FgClass.vi"("Set (F)"=TRUE, "Class In"=w515) -> ("Class Out"=w508:refnum<class "ScopePluginsBase.lvclass">)  [unwired: 9 in]
                n182 = call "Enqueue.vi"("EnqueueType (QMH)"=QueueNames."Class ", "EnqueueType (Enqueue)"=EnqueueTypes."LossyEnqueue", "error in (no error)"=w510, "Message Data"=w508, "Queue Array Reference In"=w507) -> ("error out"=w509:errorcluster)  [unwired: 4 in, 2 out]
                n183 = Path To String(path=w518) -> (string=w522:string)
                n184 = Format Into String(format string="Plugin %s loaded ", error in=w509, w522) -> (resulting string=w521:string, error out=w513:errorcluster)  [unwired: 1 in]
                n185 = call "StatusUpdate.vi"("error in (no error)"=w513, "Status"=w521, "ModuleAdmin"=w519) -> ("error out"=w520:errorcluster)  [unwired: 8 in]
              }
            }
          }
          frame "SetExtAquisition" {
            w527 = QueueNames."Class " ("EnqueueType (QMH)")
            n186 = Variant To Data(error in=w544, type=T8 {"SamplingMode "=enum."Real Time", "Interpolation"=enum."No Interpolation", "NumAverages"=8, "EnableAveraging"=FALSE, "Resolution"=enum."Auto"} ("ExtAcquisition"), Variant=w545) -> (data=w532:T8, error out=w539:errorcluster)
            n187 = call "Dequeue.vi"("EnqueueType (QMH)"=w527, "error in (no error)"=w539, "Queue Array Reference In"=w538) -> ("error out"=w537:errorcluster, "Message Data"=w536:variant, "Queue Array Reference Out"=w529:refnum<queue>[])  [unwired: 4 in, 2 out]
            n188 = call "FgClass.vi"() -> ("Class Out"=w535:refnum<class "ScopePluginsBase.lvclass">)  [unwired: 11 in]
            n189 = Variant To Data(error in=w537, type=w535, Variant=w536) -> (data=w534:refnum<class "ScopePluginsBase.lvclass">, error out=w533:errorcluster)
            n190 = call-dynamic "SetExtAcquisition.vi"("error in (no error)"=w533, "ExtAcquisition"=w532, "ScopePluginsBase in"=w534) -> ("error out"=w531:errorcluster, "ScopePluginsBase out"=w541:refnum<class "ScopePluginsBase.lvclass">)  [unwired: 7 in]
            n191 = call "FgClass.vi"("Set (F)"=TRUE, "Class In"=w541) -> ("Class Out"=w530:refnum<class "ScopePluginsBase.lvclass">)  [unwired: 9 in]
            n192 = call "Enqueue.vi"("EnqueueType (QMH)"=w527, "EnqueueType (Enqueue)"=EnqueueTypes."LossyEnqueue", "error in (no error)"=w531, "Message Data"=w530, "Queue Array Reference In"=w529) -> ("error out"=w528:errorcluster)  [unwired: 4 in, 2 out]
          }
          frame "ConfigAcquisition" {
            w546 = QueueNames."Class " ("EnqueueType (QMH)")
            n193 = call "Dequeue.vi"("EnqueueType (QMH)"=w546, "error in (no error)"=w555, "Queue Array Reference In"=w554) -> ("error out"=w558:errorcluster, "Message Data"=w557:variant, "Queue Array Reference Out"=w549:refnum<queue>[])  [unwired: 4 in, 2 out]
            n194 = call "FgClass.vi"() -> ("Class Out"=w556:refnum<class "ScopePluginsBase.lvclass">)  [unwired: 11 in]
            n195 = Variant To Data(error in=w558, type=w556, Variant=w557) -> (data=w553:refnum<class "ScopePluginsBase.lvclass">, error out=w552:errorcluster)
            n196 = call-dynamic "ConfigureAcquisition.vi"("error in (no error)"=w552, "ScopePluginsBase in"=w553) -> ("error out"=w550:errorcluster, "ScopePluginsBase out"=w561:refnum<class "ScopePluginsBase.lvclass">)  [unwired: 8 in]
            n197 = call "FgClass.vi"("Set (F)"=TRUE, "Class In"=w561) -> ("Class Out"=w548:refnum<class "ScopePluginsBase.lvclass">)  [unwired: 9 in]
            n198 = call "Enqueue.vi"("EnqueueType (QMH)"=w546, "EnqueueType (Enqueue)"=EnqueueTypes."LossyEnqueue", "error in (no error)"=w550, "Message Data"=w548, "Queue Array Reference In"=w549) -> ("error out"=w547:errorcluster)  [unwired: 4 in, 2 out]
            n199 = call "StatusUpdate.vi"("error in (no error)"=w547, "Status"="Acquisition Configured", "ModuleAdmin"=w563) -> ("error out"=w562:errorcluster)  [unwired: 8 in]
          }
          frame "ConfigChannels" {
            w567 = QueueNames."Class " ("EnqueueType (QMH)")
            n200 = call "Dequeue.vi"("EnqueueType (QMH)"=w567, "error in (no error)"=w573, "Queue Array Reference In"=w572) -> ("error out"=w576:errorcluster, "Message Data"=w575:variant, "Queue Array Reference Out"=w564:refnum<queue>[])  [unwired: 4 in, 2 out]
            n201 = call "FgClass.vi"() -> ("Class Out"=w574:refnum<class "ScopePluginsBase.lvclass">)  [unwired: 11 in]
            n202 = Variant To Data(error in=w576, type=w574, Variant=w575) -> (data=w571:refnum<class "ScopePluginsBase.lvclass">, error out=w570:errorcluster)
            n203 = call-dynamic "ConfigureChannels.vi"("error in (no error)"=w570, "ScopePluginsBase in"=w571) -> ("error out"=w568:errorcluster, "ScopePluginsBase out"=w579:refnum<class "ScopePluginsBase.lvclass">)  [unwired: 8 in]
            n204 = call "FgClass.vi"("Set (F)"=TRUE, "Class In"=w579) -> ("Class Out"=w565:refnum<class "ScopePluginsBase.lvclass">)  [unwired: 9 in]
            n205 = call "Enqueue.vi"("EnqueueType (QMH)"=w567, "EnqueueType (Enqueue)"=EnqueueTypes."LossyEnqueue", "error in (no error)"=w568, "Message Data"=w565, "Queue Array Reference In"=w564) -> ("error out"=w566:errorcluster)  [unwired: 4 in, 2 out]
            n206 = call "StatusUpdate.vi"("error in (no error)"=w566, "Status"="Channels Configured", "ModuleAdmin"=w581) -> ("error out"=w580:errorcluster)  [unwired: 8 in]
          }
          frame "SetSync" {
            w585 = QueueNames."Class " ("EnqueueType (QMH)")
            n207 = Variant To Data(error in=w603, type=T9 {"Handle"="", "SrcTerm"="", "DestTerm"=""} ("Sync"), Variant=w602) -> (data=w600:T9, error out=w591:errorcluster)
            n208 = call "Dequeue.vi"("EnqueueType (QMH)"=w585, "error in (no error)"=w591, "Queue Array Reference In"=w584) -> ("error out"=w594:errorcluster, "Message Data"=w593:variant, "Queue Array Reference Out"=w582:refnum<queue>[])  [unwired: 4 in, 2 out]
            n209 = call "FgClass.vi"() -> ("Class Out"=w592:refnum<class "ScopePluginsBase.lvclass">)  [unwired: 11 in]
            n210 = Variant To Data(error in=w594, type=w592, Variant=w593) -> (data=w589:refnum<class "ScopePluginsBase.lvclass">, error out=w590:errorcluster)
            n211 = property class="ScopePluginsBase.lvclass"(reference=w589, error in=w590, "Accessors:Sync"=w600) -> (reference out=w599:refnum<class "ScopePluginsBase.lvclass">, error out=w587:errorcluster)
            n212 = call "FgClass.vi"("Set (F)"=TRUE, "Class In"=w599) -> ("Class Out"=w583:refnum<class "ScopePluginsBase.lvclass">)  [unwired: 9 in]
            n213 = call "Enqueue.vi"("EnqueueType (QMH)"=w585, "EnqueueType (Enqueue)"=EnqueueTypes."LossyEnqueue", "error in (no error)"=w587, "Message Data"=w583, "Queue Array Reference In"=w582) -> ("error out"=w586:errorcluster)  [unwired: 4 in, 2 out]
            n214 = call "StatusUpdate.vi"("error in (no error)"=w586, "Status"="SyncInfo Set", "ModuleAdmin"=w597) -> ("error out"=w596:errorcluster)  [unwired: 8 in]
          }
          frame "ConfigTrigger" {
            w612 = QueueNames."Class " ("EnqueueType (QMH)")
            n215 = call "Dequeue.vi"("EnqueueType (QMH)"=w612, "error in (no error)"=w605, "Queue Array Reference In"=w611) -> ("error out"=w615:errorcluster, "Message Data"=w614:variant, "Queue Array Reference Out"=w604:refnum<queue>[])  [unwired: 4 in, 2 out]
            n216 = call "FgClass.vi"() -> ("Class Out"=w613:refnum<class "ScopePluginsBase.lvclass">)  [unwired: 11 in]
            n217 = Variant To Data(error in=w615, type=w613, Variant=w614) -> (data=w609:refnum<class "ScopePluginsBase.lvclass">, error out=w610:errorcluster)
            n218 = call-dynamic "ConfigureTrigger.vi"("error in (no error)"=w610, "ScopePluginsBase in"=w609) -> ("error out"=w608:errorcluster, "ScopePluginsBase out"=w607:refnum<class "ScopePluginsBase.lvclass">)  [unwired: 8 in]
            n219 = call "FgClass.vi"("Set (F)"=TRUE, "Class In"=w607) -> ("Class Out"=w616:refnum<class "ScopePluginsBase.lvclass">)  [unwired: 9 in]
            n220 = call "Enqueue.vi"("EnqueueType (QMH)"=w612, "EnqueueType (Enqueue)"=EnqueueTypes."LossyEnqueue", "error in (no error)"=w608, "Message Data"=w616, "Queue Array Reference In"=w604) -> ("error out"=w606:errorcluster)  [unwired: 4 in, 2 out]
            n221 = call "StatusUpdate.vi"("error in (no error)"=w606, "Status"="Trigger Configured", "ModuleAdmin"=w619) -> ("error out"=w621:errorcluster)  [unwired: 8 in]
          }
          frame "StartAcquisition" {
            n222 = call "FgState.vi"("Set (F)"=TRUE, "State In"="start") -> ("State Out"=w625:string)  [unwired: 9 in]
            n223 = call "Enqueue.vi"("EnqueueType (QMH)"=QueueNames."MA", "EnqueueType (Enqueue)"=EnqueueTypes."LossyEnqueue", "error in (no error)"=w627, "Message"=w625, "Queue Array Reference In"=w624) -> ("error out"=w622:errorcluster)  [unwired: 4 in, 2 out]
          }
          frame "StopAcquisition" {
            n224 = call "FgState.vi"("Set (F)"=TRUE, "State In"="stop") -> ("State Out"=w634:string)  [unwired: 9 in]
            n225 = call "Enqueue.vi"("EnqueueType (QMH)"=QueueNames."MA", "EnqueueType (Enqueue)"=EnqueueTypes."LossyEnqueue", "error in (no error)"=w636, "Message"=w634, "Queue Array Reference In"=w633) -> ("error out"=w631:errorcluster)  [unwired: 4 in, 2 out]
          }
          frame "InitScope" {
            w647 = QueueNames."Class " ("EnqueueType (QMH)")
            n226 = Variant To Data(error in=w662, type=cluster{"Reset":bool, "IdQuery":bool} {"Reset"=FALSE, "IdQuery"=FALSE}, Variant=w663) -> (data=w643:cluster{"Reset":bool, "IdQuery":bool}, error out=w646:errorcluster)
            n227 = call "Dequeue.vi"("EnqueueType (QMH)"=w647, "error in (no error)"=w646, "Queue Array Reference In"=w645) -> ("error out"=w650:errorcluster, "Message Data"=w649:variant, "Queue Array Reference Out"=w641:refnum<queue>[])  [unwired: 4 in, 2 out]
            n228 = call "FgClass.vi"() -> ("Class Out"=w648:refnum<class "ScopePluginsBase.lvclass">)  [unwired: 11 in]
            n229 = Variant To Data(error in=w650, type=w648, Variant=w649) -> (data=w642:refnum<class "ScopePluginsBase.lvclass">, error out=w644:errorcluster)
            n230 = Unbundle By Name(w643) -> ("IdQuery"=w661:bool, "Reset"=w660:bool)
            n231 = call-dynamic "Initialize.vi"("error in (no error)"=w644, "Reset (f)"=w660, "IdQuery (f)"=w661, "ScopePluginsBase in"=w642) -> ("error out"=w653:errorcluster, "ScopePluginsBase out"=w656:refnum<class "ScopePluginsBase.lvclass">)  [unwired: 6 in]
            n232 = call "FgClass.vi"("Set (F)"=TRUE, "Class In"=w656) -> ("Class Out"=w651:refnum<class "ScopePluginsBase.lvclass">)  [unwired: 9 in]
            n233 = call "Enqueue.vi"("EnqueueType (QMH)"=w647, "EnqueueType (Enqueue)"=EnqueueTypes."LossyEnqueue", "error in (no error)"=w653, "Message Data"=w651, "Queue Array Reference In"=w641) -> ("error out"=w652:errorcluster)  [unwired: 4 in, 2 out]
            n234 = call "StatusUpdate.vi"("error in (no error)"=w652, "Status"="O'Scope hardware initialized", "ModuleAdmin"=w659) -> ("error out"=w658:errorcluster)  [unwired: 8 in]
          }
          frame "Error" {
            n235 = property class="ModuleAdmin.lvclass"(reference=w670, error in=w669) -> (reference out=w667:refnum<class "ModuleAdmin.lvclass">, error out=w668:errorcluster, "Accessors:External Launch"=w674:bool, "Accessors:Module ID"=w672:i32)
            n236 = Variant To Data(error in=w668, type=errorcluster {"status"=FALSE, "code"=0, "source"=""} ("error constant"), Variant=w678) -> (data=w673:errorcluster, error out=w676:errorcluster)
            n237 = call "ReportError.vi"("error in (no error)"=w676, "ErrorReported"=w673, "ModuleID"=w672) -> ("error out"=w675:errorcluster)  [unwired: 8 in]
            n238 = case shown="True" w674 {
              tunnel: w675 -> [w681 w689]
              tunnel: w673 -> [w679 _]
              tunnel: [w681 w689] -> w671
              tunnel: w667 -> [w686 w688]
              tunnel: [w686 w688] -> w666
              tunnel: [w680 FALSE ("T button?")] -> w665
              frame False {
                w685 = T12 0 items=["no dialog", "OK message", "continue or stop message", "OK message + warnings", "continue/stop + warnings"] ("type of dialog (OK msg:1)")
                # "Stand alone: now, force an exit.Todo:  Add an event to ask the user\nIf the module should stop or continue"
                n239 = call <vilib>:"Simple Error Handler.vi"("type of dialog (OK msg:1)"=w685, "error in (no error)"=w679) -> ("message"=w682:string)  [unwired: 3 in, 4 out]
                n240 = Two Button Dialog(message=w682, 1:"Continue" ("F button name (\"Cancel\")"), 2:"Exit" ("T button name (\"OK\")")) -> (T button?=w680:bool)
              }
              frame True {
                # "Externally launched modules only broadcast the error msg"
              }
            }
            n241 = call <extravilib>:"Write.vi"("element"=w665) -> ("channel"=w664:T11)  [unwired: 1 out]
          }
          frame "QueueError" {
            w693 = TRUE
            n242 = property class="ModuleAdmin.lvclass"(reference=w697) -> (reference out=w696:refnum<class "ModuleAdmin.lvclass">, error out=w695:errorcluster, "Accessors:Module ID"=w698:i32)  [unwired: 1 in]
            n243 = call "ReportError.vi"("error in (no error)"=w695, "ErrorReported"=w692, "ModuleID"=w698) -> ("error out"=w694:errorcluster)  [unwired: 8 in]
            n244 = Merge Errors(w694, w692) -> (w691:errorcluster)
            n245 = call <extravilib>:"Write.vi"("element"=w693) -> ("channel"=w690:T11)  [unwired: 1 out]
          }
          frame "QueueTimeoutError" {
            n246 = call <extravilib>:"Read.vi"("channel"=w700) -> ("element"=w699:bool)  [unwired: 1 in, 1 out]
          }
          frame "Close" {
            w705 = QueueNames."Class " ("EnqueueType (QMH)")
            n247 = while {
              tunnel: [w726] -> w712
              tunnel: w718 -> [w727]
              tunnel: w716 -> [w725]
              tunnel: [w723] -> w711
              stop <- w730 stop-if-true
              n248 = call "Dequeue.vi"("EnqueueType (QMH)"=QueueNames."MA", "DequeueType (PreviewQueue)"=DequeueTypes."PreviewQueue", "error in (no error)"=w727, "Queue Array Reference In"=w725) -> ("error out"=w726:errorcluster, "Message"=w724:string, "Queue Array Reference Out"=w723:refnum<queue>[])  [unwired: 3 in, 2 out]
              n249 = call "FgState.vi"() -> ()  [unwired: 11 in, 1 out]
              n250 = Equal?(x=w724, y="idle") -> (x = y?=w730:bool)
            }
            n251 = call "Dequeue.vi"("EnqueueType (QMH)"=w705, "error in (no error)"=w712, "Queue Array Reference In"=w711) -> ("error out"=w715:errorcluster, "Message Data"=w714:variant, "Queue Array Reference Out"=w703:refnum<queue>[])  [unwired: 4 in, 2 out]
            n252 = call "FgClass.vi"() -> ("Class Out"=w710:refnum<class "ScopePluginsBase.lvclass">)  [unwired: 11 in]
            n253 = Variant To Data(error in=w715, type=w710, Variant=w714) -> (data=w709:refnum<class "ScopePluginsBase.lvclass">, error out=w713:errorcluster)
            n254 = call-dynamic "Close.vi"("error in (no error)"=w713, "ScopePluginsBase in"=w709) -> ("error out"=w707:errorcluster, "ScopePluginsBase out"=w722:refnum<class "ScopePluginsBase.lvclass">)  [unwired: 8 in]
            n255 = call "FgClass.vi"("Set (F)"=TRUE, "Class In"=w722) -> ("Class Out"=w704:refnum<class "ScopePluginsBase.lvclass">)  [unwired: 9 in]
            n256 = call "Enqueue.vi"("EnqueueType (QMH)"=w705, "EnqueueType (Enqueue)"=EnqueueTypes."LossyEnqueue", "error in (no error)"=w707, "Message Data"=w704, "Queue Array Reference In"=w703) -> ("error out"=w706:errorcluster)  [unwired: 4 in, 2 out]
            n257 = call "StatusUpdate.vi"("error in (no error)"=w706, "Status"="O'Scope Disconnected", "ModuleAdmin"=w721) -> ("error out"=w719:errorcluster)  [unwired: 8 in]
          }
          frame "Exit" {
            w747 = TRUE
            # "Called by the StopRequest event handler case"
            n258 = call "FgState.vi"("Set (F)"=TRUE, "State In"="exit") -> ("State Out"=w736:string)  [unwired: 9 in]
            n259 = call "Enqueue.vi"("EnqueueType (QMH)"=QueueNames."MA", "EnqueueType (Enqueue)"=EnqueueTypes."LossyEnqueue", "error in (no error)"=w734, "Message"=w736, "Queue Array Reference In"=w733) -> ("error out"=w735:errorcluster)  [unwired: 4 in, 2 out]
            n260 = control-ref of="This VI"() -> (w745:refnum<vi>)
            n261 = call "HandleExit.vi"("error in (no error)"=w735, "VI Refnum"=w745, "StopArgument"=w741, "ModuleAdmin"=w742) -> ("error out"=w746:errorcluster, "Exit via Stop Module Req?"=w743:bool, "WaitForStop?"=w744:bool)  [unwired: 5 in]
            n262 = call <extravilib>:"Write.vi"("element"=w747) -> ("channel"=w732:T11)  [unwired: 1 out]
          }
          frame Default {
            # "Called only if a message was queued and no QMH case was created"
            n263 = property class="ModuleAdmin.lvclass"(reference=w757, error in=w748) -> (reference out=w752:refnum<class "ModuleAdmin.lvclass">, error out=w749:errorcluster, "Accessors:Module ID"=w756:i32, "Accessors:ModuleName"=w753:string)
            n264 = call <userlib>:"ModuleName.vi"("Name"=w753, "ModuleID"=w756) -> ("ModuleName"=w755:string)  [unwired: 9 in]
            n265 = xnode "Error Ring"("parameter 0"=w754, "parameter 1"=w755) -> ("error out"=w751:errorcluster)
            n266 = Merge Errors(w751, w749) -> (w750:errorcluster)
          }
        }
        n267 = call "ErrorHandler.vi"("EnqueueType (QMH)"=QueueNames."QMH", "error in (no error)"=w406, "Queue Array Reference In"=w399) -> ("error out"=w407:errorcluster)  [unwired: 8 in]
        "QMH Loop" <- w400
      }
    }
    frame Error {
      n268 = property class="ModuleAdmin.lvclass"(reference=w771) -> (reference out=w770:refnum<class "ModuleAdmin.lvclass">, "Accessors:CloneRegRef"=w769:refnum<data-value>, "Accessors:Module ID"=w768:i32)  [unwired: 1 in, 1 out]
      n269 = call <userlib>:"Remove.vi"("Module ID"=w768, "CloneRegRef"=w769) -> ("error out"=w772:errorcluster)  [unwired: 7 in, 2 out]
      n270 = flat-sequence {
        tunnel: w773 -> [w776]
        tunnel: w772 -> [_]
        tunnel: [w774] -> w767
        frame #0 {
          w775 = T12 2 items=["no dialog", "OK message", "continue or stop message", "OK message + warnings", "continue/stop + warnings"] ("type of dialog (OK msg:1)")
          n271 = call <vilib>:"Simple Error Handler.vi"("type of dialog (OK msg:1)"=w775, "error in (no error)"=w776) -> ("error out"=w774:errorcluster)  [unwired: 3 in, 4 out]
        }
      }
    }
  }
  n272 = call "DestroyClone.vi"("error in (no error)"=w39, "Exit via Stop Module Req?"=w35, "Wait for Module to stop?"=w36, "ModuleAdmin"=w37) -> ("error out"=w38:errorcluster, "External Launch"=w34:bool)  [unwired: 5 in, 1 out]
  n273 = Unregister For Events(event registration refnum=w2) -> (error out=w1:errorcluster)  [unwired: 1 in]
  n274 = Release Queue(queue=w8, error in (no error)=w38) -> (error out=w24:errorcluster)  [unwired: 1 in, 2 out]
  n275 = Release Queue(queue=w7, error in (no error)=w24) -> (error out=w23:errorcluster)  [unwired: 1 in, 2 out]
  n276 = Release Queue(queue=w6, error in (no error)=w23) -> (error out=w22:errorcluster)  [unwired: 1 in, 2 out]
  n277 = case shown="True" w34 {
    tunnel: w22 -> [w777 w780]
    tunnel: [w777 w778] -> w29
    frame False {
    }
    frame True {
      n278 = control-ref of="This VI"() -> (w779:refnum<vi>)
      n279 = case shown="Error" w780 {
        selector: w780 -> [w782 _]
        tunnel: w779 -> [w783 w785]
        tunnel: [w781 w784] -> w778
        frame No Error {
          n280 = invoke class="VI" method="FP.Close"(reference=w783, error in=w782) -> (error out=w781:errorcluster)  [unwired: 1 in, 2 out]
        }
        frame Error {
          n281 = invoke class="VI" method="FP.Open"(reference=w785, "Activate"=TRUE ("Activate?")) -> (error out=w784:errorcluster)  [unwired: 3 in, 4 out]
        }
      }
    }
  }
  n282 = Merge Errors(w1, w11, w29, w30) -> (→"error out":errorcluster)
